vi "Created Aliases.vi"(11 "Base Actor in":refnum<class "Base Actor.lvclass">) -> (2 "Created Aliases":T1)   [LabVIEW 2020, in "jettl.lvlib" / "Actor.lvlib" / "Base Actor.lvclass"]
uses:
  Base Actor.lvclass
  Created Aliases.ctl
  Actor.lvlib
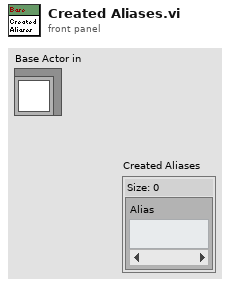
[diagram p1: front panel]
types:
  T1 = typedef "jettl.lvlib/Actor.lvlib/Created Aliases.ctl" = set{string}
  T2 = typedef "jettl.lvlib/Actor.lvlib/Alias to Created Attributes.ctl" = map{string, T3}
  T3 = typedef "jettl.lvlib/Actor.lvlib/Attributes.ctl" = cluster{"Alias":string, "Address":refnum<user-event>, "Implemented Msgs":T4, "Path":path}
  T4 = typedef "jettl.lvlib/Actor.lvlib/Implemented Msgs.ctl" = set{refnum<class "Msg.lvclass">}
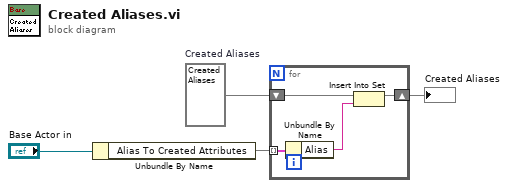
[diagram p0: block diagram]
diagram:
  w3 = T1 {}  # Created Aliases
  n1 = Unbundle By Name("Base Actor in") -> ("Alias To Created Attributes"=w1:T2)
  n2 = for {
    shift-right: [w7] -> w2
    shift-left: w3 -> [w8]
    tunnel: w1 -> [w5] mode=indexing
    n3 = Unbundle By Name(w5) -> ("Alias"=w6:string)
    n4 = Insert Into Set(10:w6, 11:w8) -> (3:w7:T1)  [unwired: 1 out]
  }
  "Created Aliases" <- w2
